vi "move_5b.vi"(6 "Array in":i32[](array[numeric]), 9 "Array 6":i32[](array[numeric]), 10 "Array 3":i32[](array[numeric]), 11 "Enum in":enum16{"move4", "move4_1", "move4_2"}(ring)) -> (1 "Array 5":i32[](array[numeric]), 2 "Array 4":i32[](array[numeric]), 3 "Enum out":T1(ring), 4 "Array out":i32[](array[numeric]))   [LabVIEW 2016]
uses:
  <vilib>/NXT/Block Support/NXT_OutputPort.ctl
  <vilib>/NXT/NXTIO Xnodes/NXTIONodeSubVIs/NXTStopMotors.vi
  <vilib>/NXT/NXTIO Xnodes/NXTIONodeSubVIs/NXTMotorRunDistance.vi
  <vilib>/NXT/NXTIO Xnodes/NXTIONodeSubVIs/LEGOMotorStatus.vi
  <vilib>/NXT/NXTIO Xnodes/NXTIONodeSubVIs/NXTMoveMotors.vi
  <vilib>/NXT/NXTIO Xnodes/NXTIONodeSubVIs/LEGOResetMotors.vi
  <vilib>/NXT/Subs/LVHSConnector.ctl
  <vilib>/NXT/NXTIO Xnodes/AddressXNode/NXTIOAddress.xnode
  <vilib>/NXT/NXTIO Xnodes/NXTIOXNode/NXTIO.xnode
  <vilib>/NXT/LegoClasses/BrickReference/BrickReference.lvclass
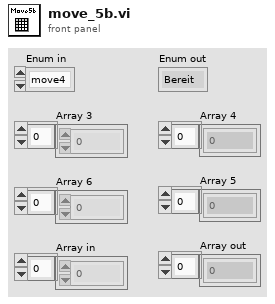
[diagram p1: front panel]
types:
  T1 = enum16{"Bereit", "Move 1", "Reference_pos", "Wait", "row1_check", "row2_check", "row3_check", "return", "move2", "move3", "move4", "move5", "end"}
  T2 = enum16{"forward", "mark", "pause", "up", "return", "end"}
  T3 = typedef "NXT_OutputPort.ctl" = u8
  T4 = cluster{"Output Port":T3, "Output Port 2":T3, "Output Port 3":T3}
  T5 = enum16{"forward", "right", "mark", "pause", "up", "return", "end"}
  T6 = typedef "LVHSConnector.ctl" = refnum<class "BrickReference.lvclass">
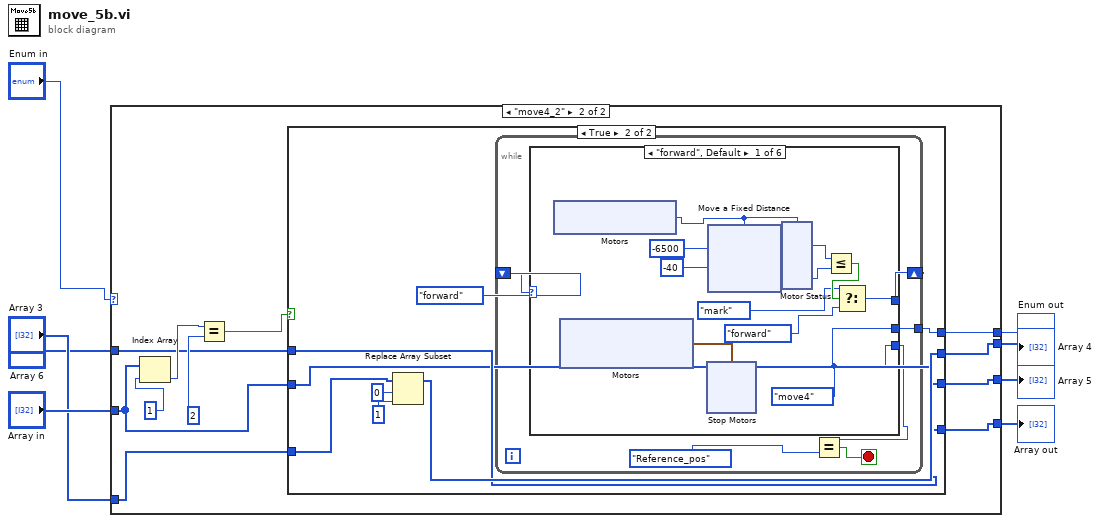
[diagram p0: block diagram]
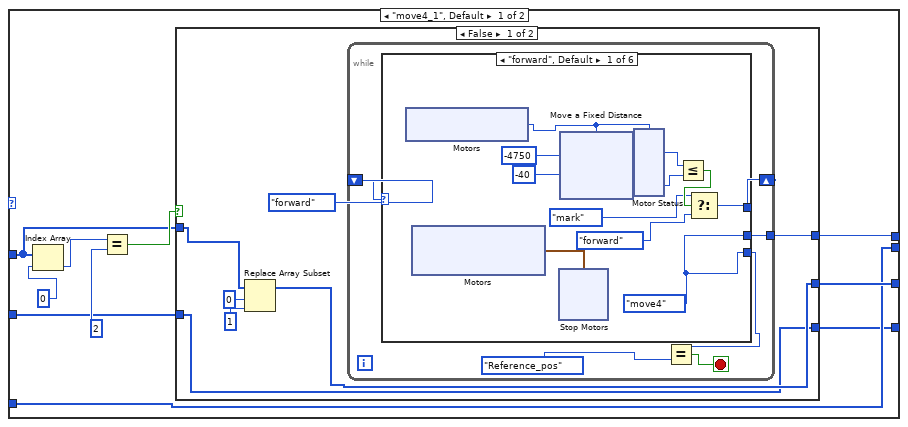
[diagram p2: hidden frame]
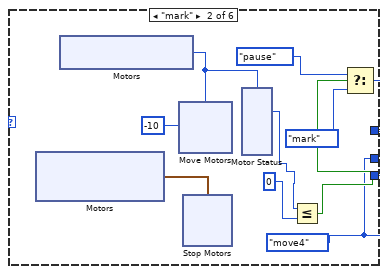
[diagram p3: hidden frame]
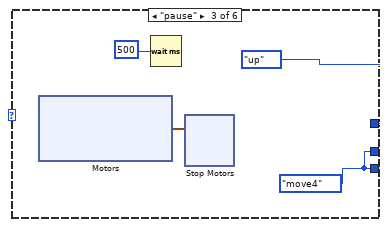
[diagram p4: hidden frame]
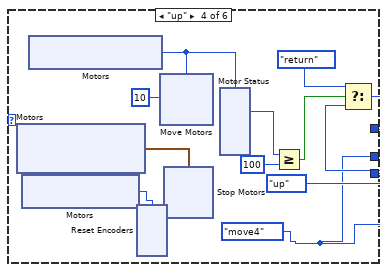
[diagram p5: hidden frame]
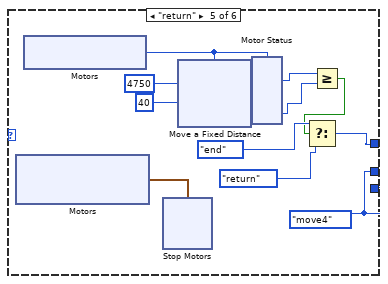
[diagram p6: hidden frame]
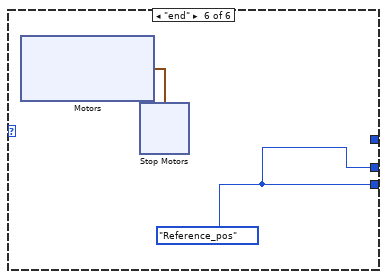
[diagram p7: hidden frame]
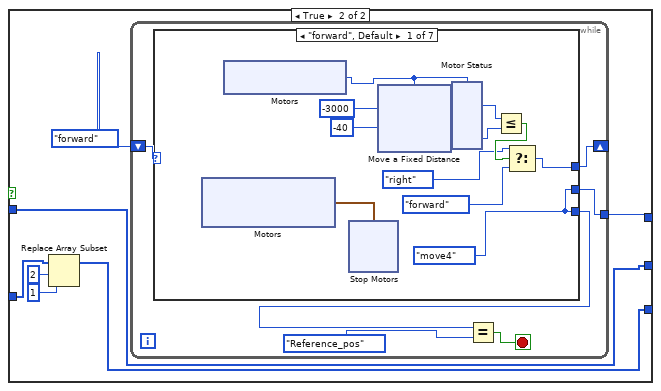
[diagram p8: hidden frame]
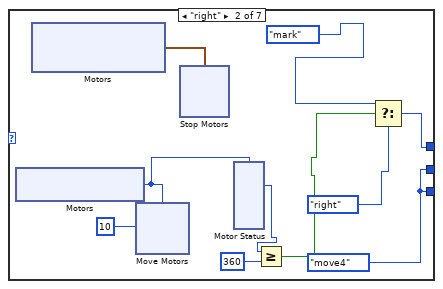
[diagram p9: hidden frame]
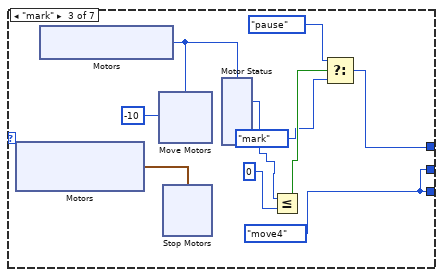
[diagram p10: hidden frame]
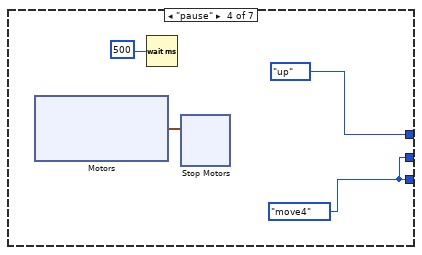
[diagram p11: hidden frame]
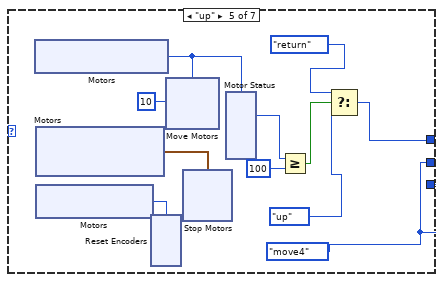
[diagram p12: hidden frame]
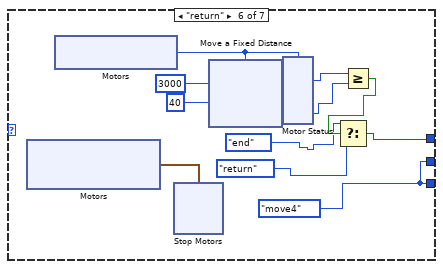
[diagram p13: hidden frame]
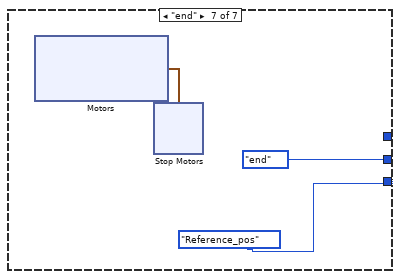
[diagram p14: hidden frame]
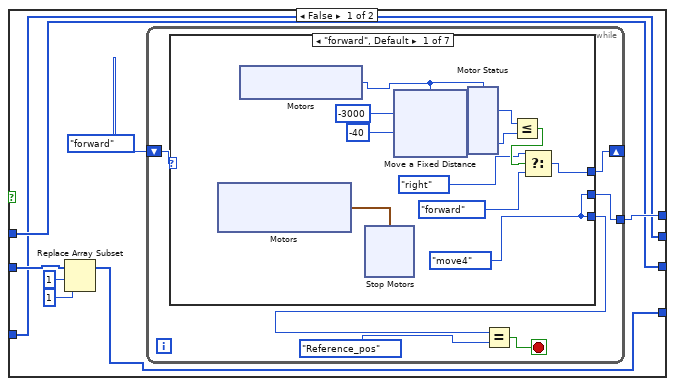
[diagram p15: hidden frame]
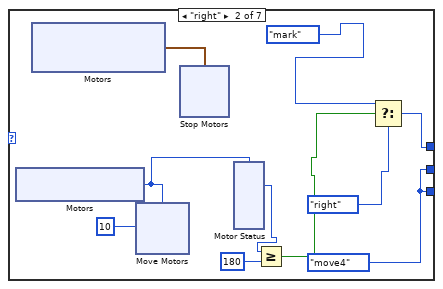
[diagram p16: hidden frame]
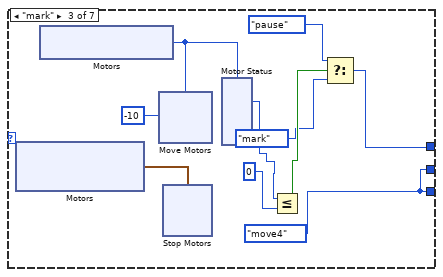
[diagram p17: hidden frame]
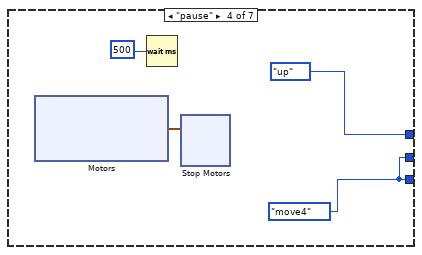
[diagram p18: hidden frame]
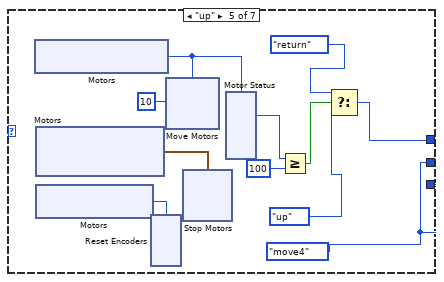
[diagram p19: hidden frame]
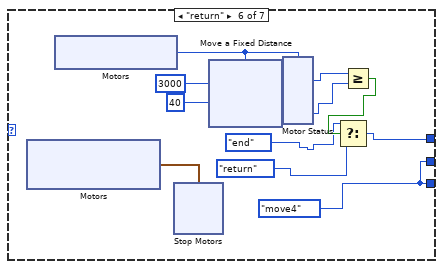
[diagram p20: hidden frame]
diagram:
  n1 = case shown="\"move4_2\"" "Enum in" {
    tunnel: [w12 w405] -> w2
    tunnel: "Array 6" -> [w14 w400]
    tunnel: [w13 w401] -> w4
    tunnel: [w11 w399] -> w5
    tunnel: "Array 3" -> [w11 w398]
    tunnel: "Array in" -> [w10 w403]
    tunnel: [w9 w402] -> w8
    frame "move4_1", Default {
      n2 = Index Array(array=w14, index=0) -> (element=w15:i32)
      n3 = Equal?(x=w15, y=2 ("element")) -> (x = y?=w17:bool)
      n4 = case shown="False" w17 {
        tunnel: w14 -> [w22 w193]
        tunnel: [w21 w193] -> w13
        tunnel: [w20 w192] -> w12
        tunnel: w10 -> [w19 w195]
        tunnel: [w19 w194] -> w9
        frame False {
          n5 = Replace Array Subset(array=w22, new element=1 ("new element/subarray"), index=0) -> (w21:i32[])
          n6 = while {
            shift-right: [w31] -> _
            shift-left: T2."forward" -> [w30]
            tunnel: [w26] -> w20
            stop <- w28 stop-if-true
            n7 = case shown="\"forward\", Default" w30 {
              tunnel: [w32 w75 T2."up" w117 w149 _] -> w31
              tunnel: [w41 w68 w100 w111 w157 w184] -> w29
              tunnel: [w41 w68 w100 w111 w157 w184] -> w26
              frame "forward", Default {
                w37 = -4750 ("Distance 1")
                w41 = T1."move4"
                n8 = xnode "Motors"() -> ("Motor"=w36:T3)
                n9 = xnode "Motors"() -> ("Motor"=w42:cluster{"Port":T3, "Port":T3})
                n10 = xnode "Stop Motors"("Motors"=w42) -> ()  [unwired: 1 in, 1 out]
                n11 = xnode "Move a Fixed Distance"("Speed 1"=i8 -40, "Distance 1"=w37, "Motors"=w36) -> ("NXT/EV3"=w38:T6)  [unwired: 1 in]
                n12 = xnode "Motor Status"("Motors"=w36, "NXT/EV3"=w38) -> ("Position 1"=w39:i32)  [unwired: 2 out]
                n13 = Less Or Equal?(x=w39, y=w37) -> (x <= y?=w35:bool)
                n14 = Select(t=T2."mark", s=w35, f=T2."forward") -> (s? t:f=w32:T2)
              }
              frame "mark" {
                w68 = T1."move4"
                n15 = xnode "Motors"() -> ("Motor"=w77:cluster{"Port":T3, "Port":T3})
                n16 = xnode "Motors"() -> ("Motor"=w72:T3)
                n17 = xnode "Move Motors"("Power/Speed 1"=i8 -10, "Motors"=w72) -> ()  [unwired: 1 in, 1 out]
                n18 = xnode "Stop Motors"("Motors"=w77) -> ()  [unwired: 1 in, 1 out]
                n19 = xnode "Motor Status"("Motors"=w72) -> ("Position 1"=w71:i32)  [unwired: 1 in, 2 out]
                n20 = Less Or Equal?(x=w71, y=0) -> (x <= y?=w69:bool)
                n21 = Select(t=T2."pause", s=w69, f=T2."mark") -> (s? t:f=w75:T2)
              }
              frame "pause" {
                w100 = T1."move4"
                n22 = xnode "Motors"() -> ("Motor"=w103:cluster{"Port":T3, "Port":T3, "Port":T3})
                n23 = Wait (ms)(milliseconds to wait=u32 500 ("millisecond timer value")) -> ()  [unwired: 1 out]
                n24 = xnode "Stop Motors"("Motors"=w103) -> ()  [unwired: 1 in, 1 out]
              }
              frame "up" {
                w111 = T1."move4"
                n25 = xnode "Motors"() -> ("Motor"=w119:cluster{"Port":T3, "Port":T3})
                n26 = xnode "Motors"() -> ("Motor"=w110:T3)
                n27 = xnode "Motors"() -> ("Motor"=w113:T3)
                n28 = xnode "Reset Encoders"("Motors"=w110) -> ()  [unwired: 1 in, 1 out]
                n29 = xnode "Move Motors"("Power/Speed 1"=i8 10, "Motors"=w113) -> ()  [unwired: 1 in, 1 out]
                n30 = xnode "Stop Motors"("Motors"=w119) -> ()  [unwired: 1 in, 1 out]
                n31 = xnode "Motor Status"("Motors"=w113) -> ("Position 1"=w114:i32)  [unwired: 1 in, 2 out]
                n32 = Greater Or Equal?(x=w114, y=100) -> (x >= y?=w118:bool)
                n33 = Select(t=T2."return", s=w118, f=T2."up") -> (s? t:f=w117:T2)
              }
              frame "return" {
                w152 = 4750 ("Distance 1")
                w157 = T1."move4"
                n34 = xnode "Motors"() -> ("Motor"=w158:cluster{"Port":T3, "Port":T3})
                n35 = xnode "Motors"() -> ("Motor"=w155:T3)
                n36 = xnode "Stop Motors"("Motors"=w158) -> ()  [unwired: 1 in, 1 out]
                n37 = xnode "Move a Fixed Distance"("Speed 1"=i8 40, "Distance 1"=w152, "Motors"=w155) -> ("NXT/EV3"=w154:T6)  [unwired: 1 in]
                n38 = xnode "Motor Status"("Motors"=w155, "NXT/EV3"=w154) -> ("Position 1"=w153:i32)  [unwired: 2 out]
                n39 = Greater Or Equal?(x=w153, y=w152) -> (x >= y?=w148:bool)
                n40 = Select(t=T2."end", s=w148, f=T2."return") -> (s? t:f=w149:T2)
              }
              frame "end" {
                w184 = T1."Reference_pos"
                n41 = xnode "Motors"() -> ("Motor"=w185:cluster{"Port":T3, "Port":T3, "Port":T3})
                n42 = xnode "Stop Motors"("Motors"=w185) -> ()  [unwired: 1 in, 1 out]
              }
            }
            n43 = Equal?(x=w29, y=T1."Reference_pos") -> (x = y?=w28:bool)
          }
        }
        frame True {
          n44 = Replace Array Subset(array=w195, new element=1 ("new element/subarray"), index=2) -> (w194:i32[])
          n45 = while {
            shift-right: [w200] -> _
            shift-left: T5."forward" -> [w201]
            tunnel: [w199] -> w192
            stop <- w203 stop-if-true
            n46 = case shown="\"forward\", Default" w201 {
              tunnel: [w205 w242 w274 T5."up" w317 w353 _] -> w200
              tunnel: [w214 w241 w273 w305 w316 w362 T1."Reference_pos"] -> w204
              tunnel: [w214 w241 w273 w305 w316 w362 T1."end"] -> w199
              frame "forward", Default {
                w210 = -3000 ("Distance 1")
                w214 = T1."move4"
                n47 = xnode "Motors"() -> ("Motor"=w215:cluster{"Port":T3, "Port":T3})
                n48 = xnode "Motors"() -> ("Motor"=w209:T3)
                n49 = xnode "Stop Motors"("Motors"=w215) -> ()  [unwired: 1 in, 1 out]
                n50 = xnode "Move a Fixed Distance"("Speed 1"=i8 -40, "Distance 1"=w210, "Motors"=w209) -> ("NXT/EV3"=w211:T6)  [unwired: 1 in]
                n51 = xnode "Motor Status"("Motors"=w209, "NXT/EV3"=w211) -> ("Position 1"=w212:i32)  [unwired: 2 out]
                n52 = Less Or Equal?(x=w212, y=w210) -> (x <= y?=w208:bool)
                n53 = Select(t=T5."right", s=w208, f=T5."forward") -> (s? t:f=w205:T5)
              }
              frame "right" {
                w241 = T1."move4"
                n54 = xnode "Motors"() -> ("Motor"=w250:T3)
                n55 = xnode "Motors"() -> ("Motor"=w249:cluster{"Port":T3, "Port":T3})
                n56 = xnode "Move Motors"("Power/Speed 1"=i8 10, "Motors"=w250) -> ()  [unwired: 1 in, 1 out]
                n57 = xnode "Stop Motors"("Motors"=w249) -> ()  [unwired: 1 in, 1 out]
                n58 = xnode "Motor Status"("Motors"=w250) -> ("Position 1"=w247:i32)  [unwired: 1 in, 2 out]
                n59 = Greater Or Equal?(x=w247, y=360) -> (x >= y?=w246:bool)
                n60 = Select(t=T5."mark", s=w246, f=T5."right") -> (s? t:f=w242:T5)
              }
              frame "mark" {
                w273 = T1."move4"
                n61 = xnode "Motors"() -> ("Motor"=w282:cluster{"Port":T3, "Port":T3})
                n62 = xnode "Motors"() -> ("Motor"=w280:T3)
                n63 = xnode "Move Motors"("Power/Speed 1"=i8 -10, "Motors"=w280) -> ()  [unwired: 1 in, 1 out]
                n64 = xnode "Stop Motors"("Motors"=w282) -> ()  [unwired: 1 in, 1 out]
                n65 = xnode "Motor Status"("Motors"=w280) -> ("Position 1"=w279:i32)  [unwired: 1 in, 2 out]
                n66 = Less Or Equal?(x=w279, y=0) -> (x <= y?=w277:bool)
                n67 = Select(t=T5."pause", s=w277, f=T5."mark") -> (s? t:f=w274:T5)
              }
              frame "pause" {
                w305 = T1."move4"
                n68 = xnode "Motors"() -> ("Motor"=w308:cluster{"Port":T3, "Port":T3, "Port":T3})
                n69 = Wait (ms)(milliseconds to wait=u32 500 ("millisecond timer value")) -> ()  [unwired: 1 out]
                n70 = xnode "Stop Motors"("Motors"=w308) -> ()  [unwired: 1 in, 1 out]
              }
              frame "up" {
                w316 = T1."move4"
                n71 = xnode "Motors"() -> ("Motor"=w321:T3)
                n72 = xnode "Motors"() -> ("Motor"=w324:cluster{"Port":T3, "Port":T3})
                n73 = xnode "Motors"() -> ("Motor"=w315:T3)
                n74 = xnode "Reset Encoders"("Motors"=w315) -> ()  [unwired: 1 in, 1 out]
                n75 = xnode "Move Motors"("Power/Speed 1"=i8 10, "Motors"=w321) -> ()  [unwired: 1 in, 1 out]
                n76 = xnode "Stop Motors"("Motors"=w324) -> ()  [unwired: 1 in, 1 out]
                n77 = xnode "Motor Status"("Motors"=w321) -> ("Position 1"=w322:i32)  [unwired: 1 in, 2 out]
                n78 = Greater Or Equal?(x=w322, y=100) -> (x >= y?=w323:bool)
                n79 = Select(t=T5."return", s=w323, f=T5."up") -> (s? t:f=w317:T5)
              }
              frame "return" {
                w357 = 3000 ("Distance 1")
                w362 = T1."move4"
                n80 = xnode "Motors"() -> ("Motor"=w363:cluster{"Port":T3, "Port":T3})
                n81 = xnode "Motors"() -> ("Motor"=w360:T3)
                n82 = xnode "Stop Motors"("Motors"=w363) -> ()  [unwired: 1 in, 1 out]
                n83 = xnode "Move a Fixed Distance"("Speed 1"=i8 40, "Distance 1"=w357, "Motors"=w360) -> ("NXT/EV3"=w359:T6)  [unwired: 1 in]
                n84 = xnode "Motor Status"("Motors"=w360, "NXT/EV3"=w359) -> ("Position 1"=w358:i32)  [unwired: 2 out]
                n85 = Greater Or Equal?(x=w358, y=w357) -> (x >= y?=w356:bool)
                n86 = Select(t=T5."end", s=w356, f=T5."return") -> (s? t:f=w353:T5)
              }
              frame "end" {
                n87 = xnode "Motors"() -> ("Motor"=w390:cluster{"Port":T3, "Port":T3, "Port":T3})
                n88 = xnode "Stop Motors"("Motors"=w390) -> ()  [unwired: 1 in, 1 out]
              }
            }
            n89 = Equal?(x=w204, y=T1."Reference_pos") -> (x = y?=w203:bool)
          }
        }
      }
    }
    frame "move4_2" {
      n90 = Index Array(array=w403, index=1) -> (element=w404:i32)
      n91 = Equal?(x=w404, y=2 ("element")) -> (x = y?=w407:bool)
      n92 = case shown="True" w407 {
        tunnel: [w413 w620] -> w405
        tunnel: w403 -> [w412 w616]
        tunnel: [w411 w616] -> w402
        tunnel: [w410 w617] -> w401
        tunnel: w400 -> [w410 w617]
        tunnel: [w409 w618] -> w399
        tunnel: w398 -> [w409 w619]
        frame False {
          n93 = Replace Array Subset(array=w412, new element=1 ("new element/subarray"), index=1) -> (w411:i32[])
          n94 = while {
            shift-right: [w418] -> _
            shift-left: T5."forward" -> [w419]
            tunnel: [w417] -> w413
            stop <- w421 stop-if-true
            n95 = case shown="\"forward\", Default" w419 {
              tunnel: [w423 w460 w492 T5."up" w535 w571 _] -> w418
              tunnel: [w432 w459 w491 w523 w534 w580 T1."Reference_pos"] -> w422
              tunnel: [w432 w459 w491 w523 w534 w580 T1."end"] -> w417
              frame "forward", Default {
                w428 = -3000 ("Distance 1")
                w432 = T1."move4"
                n96 = xnode "Motors"() -> ("Motor"=w433:cluster{"Port":T3, "Port":T3})
                n97 = xnode "Motors"() -> ("Motor"=w427:T3)
                n98 = xnode "Stop Motors"("Motors"=w433) -> ()  [unwired: 1 in, 1 out]
                n99 = xnode "Move a Fixed Distance"("Speed 1"=i8 -40, "Distance 1"=w428, "Motors"=w427) -> ("NXT/EV3"=w429:T6)  [unwired: 1 in]
                n100 = xnode "Motor Status"("Motors"=w427, "NXT/EV3"=w429) -> ("Position 1"=w430:i32)  [unwired: 2 out]
                n101 = Less Or Equal?(x=w430, y=w428) -> (x <= y?=w426:bool)
                n102 = Select(t=T5."right", s=w426, f=T5."forward") -> (s? t:f=w423:T5)
              }
              frame "right" {
                w459 = T1."move4"
                n103 = xnode "Motors"() -> ("Motor"=w468:T3)
                n104 = xnode "Motors"() -> ("Motor"=w467:cluster{"Port":T3, "Port":T3})
                n105 = xnode "Move Motors"("Power/Speed 1"=i8 10, "Motors"=w468) -> ()  [unwired: 1 in, 1 out]
                n106 = xnode "Stop Motors"("Motors"=w467) -> ()  [unwired: 1 in, 1 out]
                n107 = xnode "Motor Status"("Motors"=w468) -> ("Position 1"=w465:i32)  [unwired: 1 in, 2 out]
                n108 = Greater Or Equal?(x=w465, y=180) -> (x >= y?=w464:bool)
                n109 = Select(t=T5."mark", s=w464, f=T5."right") -> (s? t:f=w460:T5)
              }
              frame "mark" {
                w491 = T1."move4"
                n110 = xnode "Motors"() -> ("Motor"=w500:cluster{"Port":T3, "Port":T3})
                n111 = xnode "Motors"() -> ("Motor"=w498:T3)
                n112 = xnode "Move Motors"("Power/Speed 1"=i8 -10, "Motors"=w498) -> ()  [unwired: 1 in, 1 out]
                n113 = xnode "Stop Motors"("Motors"=w500) -> ()  [unwired: 1 in, 1 out]
                n114 = xnode "Motor Status"("Motors"=w498) -> ("Position 1"=w497:i32)  [unwired: 1 in, 2 out]
                n115 = Less Or Equal?(x=w497, y=0) -> (x <= y?=w495:bool)
                n116 = Select(t=T5."pause", s=w495, f=T5."mark") -> (s? t:f=w492:T5)
              }
              frame "pause" {
                w523 = T1."move4"
                n117 = xnode "Motors"() -> ("Motor"=w526:cluster{"Port":T3, "Port":T3, "Port":T3})
                n118 = Wait (ms)(milliseconds to wait=u32 500 ("millisecond timer value")) -> ()  [unwired: 1 out]
                n119 = xnode "Stop Motors"("Motors"=w526) -> ()  [unwired: 1 in, 1 out]
              }
              frame "up" {
                w534 = T1."move4"
                n120 = xnode "Motors"() -> ("Motor"=w539:T3)
                n121 = xnode "Motors"() -> ("Motor"=w542:cluster{"Port":T3, "Port":T3})
                n122 = xnode "Motors"() -> ("Motor"=w533:T3)
                n123 = xnode "Reset Encoders"("Motors"=w533) -> ()  [unwired: 1 in, 1 out]
                n124 = xnode "Move Motors"("Power/Speed 1"=i8 10, "Motors"=w539) -> ()  [unwired: 1 in, 1 out]
                n125 = xnode "Stop Motors"("Motors"=w542) -> ()  [unwired: 1 in, 1 out]
                n126 = xnode "Motor Status"("Motors"=w539) -> ("Position 1"=w540:i32)  [unwired: 1 in, 2 out]
                n127 = Greater Or Equal?(x=w540, y=100) -> (x >= y?=w541:bool)
                n128 = Select(t=T5."return", s=w541, f=T5."up") -> (s? t:f=w535:T5)
              }
              frame "return" {
                w575 = 3000 ("Distance 1")
                w580 = T1."move4"
                n129 = xnode "Motors"() -> ("Motor"=w581:cluster{"Port":T3, "Port":T3})
                n130 = xnode "Motors"() -> ("Motor"=w578:T3)
                n131 = xnode "Stop Motors"("Motors"=w581) -> ()  [unwired: 1 in, 1 out]
                n132 = xnode "Move a Fixed Distance"("Speed 1"=i8 40, "Distance 1"=w575, "Motors"=w578) -> ("NXT/EV3"=w577:T6)  [unwired: 1 in]
                n133 = xnode "Motor Status"("Motors"=w578, "NXT/EV3"=w577) -> ("Position 1"=w576:i32)  [unwired: 2 out]
                n134 = Greater Or Equal?(x=w576, y=w575) -> (x >= y?=w574:bool)
                n135 = Select(t=T5."end", s=w574, f=T5."return") -> (s? t:f=w571:T5)
              }
              frame "end" {
                n136 = xnode "Motors"() -> ("Motor"=w608:cluster{"Port":T3, "Port":T3, "Port":T3})
                n137 = xnode "Stop Motors"("Motors"=w608) -> ()  [unwired: 1 in, 1 out]
              }
            }
            n138 = Equal?(x=w422, y=T1."Reference_pos") -> (x = y?=w421:bool)
          }
        }
        frame True {
          n139 = Replace Array Subset(array=w619, new element=1 ("new element/subarray"), index=0) -> (w618:i32[])
          n140 = while {
            shift-right: [w629] -> _
            shift-left: T2."forward" -> [w628]
            tunnel: [w624] -> w620
            stop <- w626 stop-if-true
            n141 = case shown="\"forward\", Default" w628 {
              tunnel: [w630 w673 T2."up" w715 w747 _] -> w629
              tunnel: [w639 w666 w698 w709 w755 T1."Reference_pos"] -> w627
              tunnel: [w639 w666 w698 w709 w755 T1."end"] -> w624
              frame "forward", Default {
                w635 = -6500 ("Distance 1")
                w639 = T1."move4"
                n142 = xnode "Motors"() -> ("Motor"=w634:T3)
                n143 = xnode "Motors"() -> ("Motor"=w640:cluster{"Port":T3, "Port":T3})
                n144 = xnode "Stop Motors"("Motors"=w640) -> ()  [unwired: 1 in, 1 out]
                n145 = xnode "Move a Fixed Distance"("Speed 1"=i8 -40, "Distance 1"=w635, "Motors"=w634) -> ("NXT/EV3"=w636:T6)  [unwired: 1 in]
                n146 = xnode "Motor Status"("Motors"=w634, "NXT/EV3"=w636) -> ("Position 1"=w637:i32)  [unwired: 2 out]
                n147 = Less Or Equal?(x=w637, y=w635) -> (x <= y?=w633:bool)
                n148 = Select(t=T2."mark", s=w633, f=T2."forward") -> (s? t:f=w630:T2)
              }
              frame "mark" {
                w666 = T1."move4"
                n149 = xnode "Motors"() -> ("Motor"=w675:cluster{"Port":T3, "Port":T3})
                n150 = xnode "Motors"() -> ("Motor"=w670:T3)
                n151 = xnode "Move Motors"("Power/Speed 1"=i8 -10, "Motors"=w670) -> ()  [unwired: 1 in, 1 out]
                n152 = xnode "Stop Motors"("Motors"=w675) -> ()  [unwired: 1 in, 1 out]
                n153 = xnode "Motor Status"("Motors"=w670) -> ("Position 1"=w669:i32)  [unwired: 1 in, 2 out]
                n154 = Less Or Equal?(x=w669, y=0) -> (x <= y?=w667:bool)
                n155 = Select(t=T2."pause", s=w667, f=T2."mark") -> (s? t:f=w673:T2)
              }
              frame "pause" {
                w698 = T1."move4"
                n156 = xnode "Motors"() -> ("Motor"=w701:cluster{"Port":T3, "Port":T3, "Port":T3})
                n157 = Wait (ms)(milliseconds to wait=u32 500 ("millisecond timer value")) -> ()  [unwired: 1 out]
                n158 = xnode "Stop Motors"("Motors"=w701) -> ()  [unwired: 1 in, 1 out]
              }
              frame "up" {
                w709 = T1."move4"
                n159 = xnode "Motors"() -> ("Motor"=w717:cluster{"Port":T3, "Port":T3})
                n160 = xnode "Motors"() -> ("Motor"=w708:T3)
                n161 = xnode "Motors"() -> ("Motor"=w711:T3)
                n162 = xnode "Reset Encoders"("Motors"=w708) -> ()  [unwired: 1 in, 1 out]
                n163 = xnode "Move Motors"("Power/Speed 1"=i8 10, "Motors"=w711) -> ()  [unwired: 1 in, 1 out]
                n164 = xnode "Stop Motors"("Motors"=w717) -> ()  [unwired: 1 in, 1 out]
                n165 = xnode "Motor Status"("Motors"=w711) -> ("Position 1"=w712:i32)  [unwired: 1 in, 2 out]
                n166 = Greater Or Equal?(x=w712, y=100) -> (x >= y?=w716:bool)
                n167 = Select(t=T2."return", s=w716, f=T2."up") -> (s? t:f=w715:T2)
              }
              frame "return" {
                w750 = 6500 ("Distance 1")
                w755 = T1."move4"
                n168 = xnode "Motors"() -> ("Motor"=w756:cluster{"Port":T3, "Port":T3})
                n169 = xnode "Motors"() -> ("Motor"=w753:T3)
                n170 = xnode "Stop Motors"("Motors"=w756) -> ()  [unwired: 1 in, 1 out]
                n171 = xnode "Move a Fixed Distance"("Speed 1"=i8 40, "Distance 1"=w750, "Motors"=w753) -> ("NXT/EV3"=w752:T6)  [unwired: 1 in]
                n172 = xnode "Motor Status"("Motors"=w753, "NXT/EV3"=w752) -> ("Position 1"=w751:i32)  [unwired: 2 out]
                n173 = Greater Or Equal?(x=w751, y=w750) -> (x >= y?=w746:bool)
                n174 = Select(t=T2."end", s=w746, f=T2."return") -> (s? t:f=w747:T2)
              }
              frame "end" {
                n175 = xnode "Motors"() -> ("Motor"=w784:cluster{"Port":T3, "Port":T3, "Port":T3})
                n176 = xnode "Stop Motors"("Motors"=w784) -> ()  [unwired: 1 in, 1 out]
              }
            }
            n177 = Equal?(x=w627, y=T1."Reference_pos") -> (x = y?=w626:bool)
          }
        }
      }
    }
  }
  "Array out" <- w8
  "Array 4" <- w5
  "Array 5" <- w4
  "Enum out" <- w2
